vi "Drive.vi"(0 "Robot Commands":T1, 11 "Error In":errorcluster) -> (15 "Error Out":errorcluster)   [LabVIEW 2014]
uses:
  Subsystem VIs/Robot Commands.ctl
  Global Variables/Refnum Names.vi
  <vilib>/Rock Robotics/WPI/RobotDrive/WPI_RobotDriveGetSetRefNum.vi
  <vilib>/Rock Robotics/WPI/RobotDrive/WPI_RobotDriveMecanumDrive_Cartesian.vi
  <vilib>/Rock Robotics/Network Tables/SD Write Numeric Array.vi
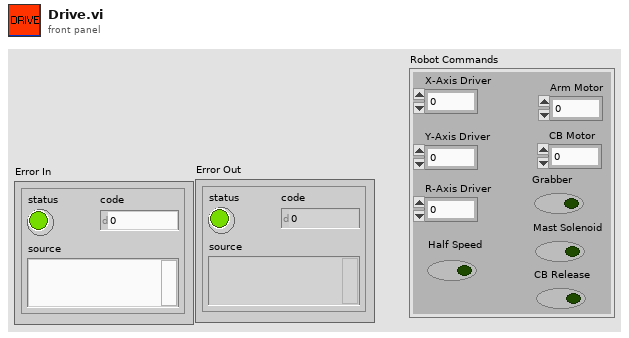
[diagram p1: front panel]
types:
  T1 = typedef "Robot Commands.ctl" = cluster{"X-Axis Driver":dbl, "Y-Axis Driver":dbl, "R-Axis Driver":dbl, "Arm Motor":dbl, "CB Motor":dbl, "Grabber":bool, "Mast Solenoid":bool, "CB Release":bool, "Half Speed":bool}
  T2 = typedef "WPI_RobotDriveDevRef.ctl" = cluster{"DevStatus":errorcluster, "Motors[]":T3[], "Square Inputs":bool, "Max Output":dbl}
  T3 = typedef "WPI_MotorControlDeviceRef.ctl" = cluster{"DeviceStatus":errorcluster, "Type":T4, "PWM":cluster{"Controller":T5, "PWM Channel":T6, "DeadBand":T7}, "CAN":cluster{"Device Number":u8, "Control Mode":T8, "Semaphore":T9, "Max Vout":dbl, "TalonSRX Control Mode":T10}, "Invert":bool, "TransformRef":T11, "InvTransformRef":T11}
  T4 = typedef "WPI_MotorControlType.ctl" = enum16{"PWM", "CAN", "CANTalonSRX"}
  T5 = typedef "FPGA_TypedefDigitalModule.ctl" = enum16{"Controller 1"}
  T6 = typedef "FPGA_DIOPWMChannel.ctl" = enum8{"PWM 0", "PWM 1", "PWM 2", "PWM 3", "PWM 4", "PWM 5", "PWM 6", "PWM 7", "PWM 8", "PWM 9", "PWM MXP 0", "PWM MXP 1", "PWM MXP 2", "PWM MXP 3", "PWM MXP 4", "PWM MXP 5", "PWM MXP 6", "PWM MXP 7", "PWM MXP 8", "PWM MXP 9", "Invalid"}
  T7 = typedef "WPI_PWMDeadband.ctl" = cluster{"Name":string, "maxPositivePwm":i32, "minPositivePwm":i32, "centerPwm":i32, "maxNegativePwm":i32, "minNegativePwm":i32, "angularRange":u16}
  T8 = typedef "WPI_CANJaguar_ControlMode.ctl" = enum8{"Percent VBus", "Current", "Speed", "Position", "Voltage"}
  T9 = typedef "Semaphore RefNum" = refnum<k1>
  T10 = typedef "WPI_CANTalonSRX_APIControlMode.ctl" = enum8{"Percent VBus", "Speed", "Position", "Slave", "Unchanged / Invalid"}
  T11 = typedef "WPI_PWMTransform_ConPane.ctl" = refnum<vi>
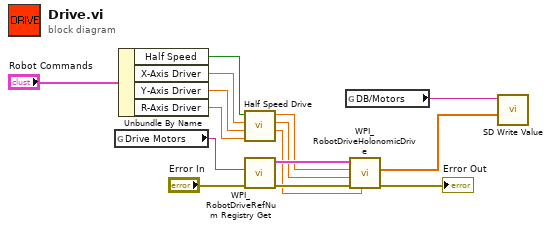
[diagram p0: block diagram]
diagram:
  n1 = global read "Refnum Names.vi" "Drive Motors"() -> (w10:string)
  n2 = Unbundle By Name("Robot Commands") -> ("Half Speed"=w1:bool, "X-Axis Driver"=w2:dbl, "Y-Axis Driver"=w3:dbl, "R-Axis Driver"=w4:dbl)
  n3 = call "Half Speed Drive.vi"("R In"=w4, "Y In"=w3, "X In"=w2, "Half Speed"=w1) -> ("R Out"=w6:dbl, "Y Out"=w7:dbl, "X Out"=w8:dbl)  [unwired: 5 in]
  n4 = call <vilib>:"WPI_RobotDriveRefNum Registry Get.vi"("error in (no error)"="Error In", "refnum name"=w10) -> ("error out"=w15:errorcluster, "RobotDriveDevRef"=w14:T2)  [unwired: 8 in]
  n5 = global read "Refnum Names.vi" "DB/Motors"() -> (w9:string)
  n6 = call-poly <vilib>:"WPI_RobotDriveHolonomicDrive.vi"("Rotation"=w6, "error in (no error)"=w15, "Y"=w7, "X"=w8, "RobotDriveDevRef"=w14) -> ("error out"=→"Error Out":errorcluster, "Motor Values"=w13:dbl[])  [unwired: 4 in, 1 out]
  n7 = call-poly <vilib>:"SD Write Value.vi"("Numeric Array"=w13, "Name"=w9) -> ()  [unwired: 8 in, 2 out]
